vi "Selection Indices.vi"(8 "error in (no error)":errorcluster, 10 "Channel Tree Tag":string, 11 "GenericGuiAO in":refnum<class "GenericGuiAO.lvclass">) -> (0 "error out":errorcluster, 3 "GenericGuiAO out":refnum<class "GenericGuiAO.lvclass">)   [LabVIEW 2020, in "VolatusDAQGenericGUI.lvlib" / "GenericGuiAO.lvclass"]
uses:
  GenericGuiAO.lvclass
  GenericGuiAO.lvclass/GenericGuiAO.ctl
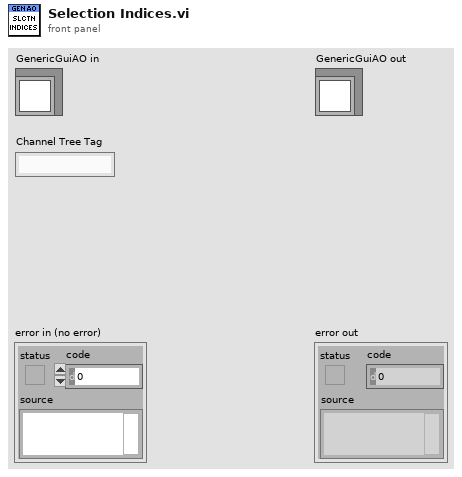
[diagram p1: front panel]
types:
  T1 = typedef "VolatusDAQGenericGUI.lvlib/Group Info.ctl" = cluster{"Group":refnum<class "Group.lvclass">, "Channel Names":string[], "Resources":string[], "Node":string, "Task":string}
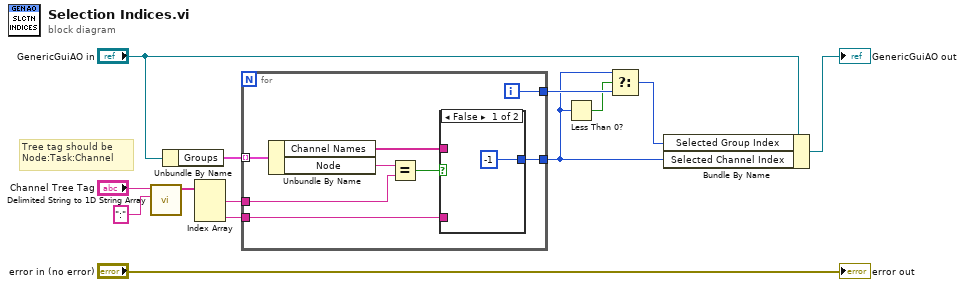
[diagram p0: block diagram]
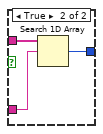
[diagram p2: hidden frame]
diagram:
  # "Tree tag should be\nNode:Task:Channel"
  n1 = call <vilib>:"Delimited String to 1D String Array.vi"("delimiter"=":", "delimited string"="Channel Tree Tag") -> ("string array"=w8:string[])  [unwired: 9 in]
  n2 = Unbundle By Name("GenericGuiAO in") -> ("Groups"=w9:T1[])
  n3 = Index Array(array=w8) -> (element #1=w7:string, element #3=w6:string)  [unwired: 3 in, 1 out]
  n4 = for {
    tunnel: w9 -> [w21] mode=indexing
    tunnel: w7 -> [w19]
    tunnel: w6 -> [w16]
    tunnel: [w15] -> w4
    tunnel: [w14] -> w2
    i -> [w15]
    n5 = Unbundle By Name(w21) -> ("Channel Names"=w17:string[], "Node"=w20:string)
    n6 = Equal?(x=w20, y=w19) -> (x = y?=w18:bool)
    n7 = case shown="False" w18 {
      tunnel: w17 -> [_ w25]
      tunnel: w16 -> [_ w24]
      tunnel: [-1 ("index of element") w23] -> w14
      frame False {
      }
      frame True {
        n8 = Search 1D Array(1D array=w25, element=w24) -> (index of element=w23:i32)  [unwired: 1 in]
      }
    }
  }
  n9 = Less Than 0?(x=w2) -> (x < 0?=w3:bool)
  n10 = Select(t=w2, s=w3, f=w4) -> (s? t:f=w1:i32)
  n11 = Bundle By Name(cluster="GenericGuiAO in", "Selected Group Index"=w1, "Selected Channel Index"=w2) -> (→"GenericGuiAO out":refnum<class "GenericGuiAO.lvclass">)
  "error out" <- "error in (no error)"
